vi "Write All Elements GUI.vi"(8 "error in (no error)":errorcluster, 10 "Correction params.":T1={"Background correction"=FALSE, "Hot-pixel correction"=FALSE, "Black image cam. 1"=path "C:/CameraVision/Black images/Black-CameraA-Full.bmp", "Black image cam. 2"=path "C:/CameraVision/Black images/Black-CameraB-Full.bmp", "Y-shift"=0, "X-shift"=0, "Correlation algorithm"=enum."Fixed shift", "Noise treshold"=25.0, "Smoothing algorithm"=enum."Noise tresholding", "2nd image correlation"=FALSE, "Image smoothing"=FALSE, "Background correction method"=enum."Hardware"} {"Noise treshold" min=0 max=255 step=1}, 11 "Correct params in":refnum<class "CV-Correction.lvclass">) -> (0 "error out":errorcluster, 3 "Correct params out":refnum<class "CV-Correction.lvclass">)   [LabVIEW 2013, in "CameraVision.lvlib" / "CV-Correction.lvclass"]
uses:
  CV-Correction.lvclass
  Correction-parameters-gui.ctl
  Smoothing.ctl
  Background-correction.ctl
  CV-Correction.lvclass/CV-Correction.ctl
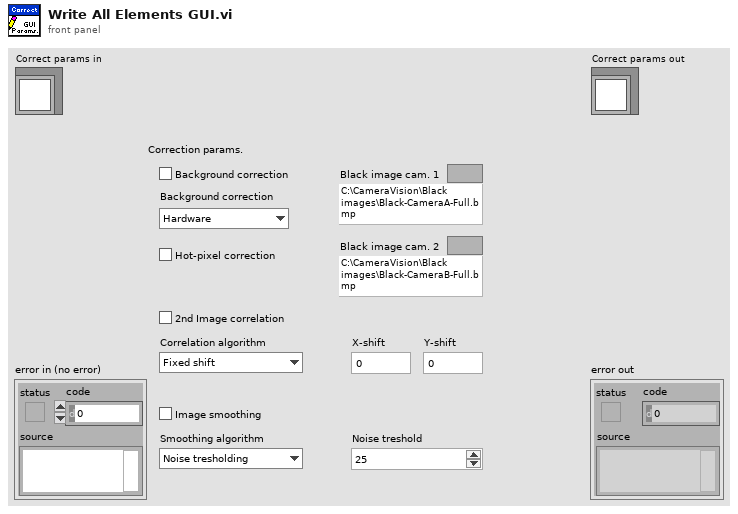
[diagram p1: front panel]
types:
  T1 = typedef "CameraVision.lvlib/CV-Correction.lvclass/Correction-parameters-gui.ctl" = cluster{"Background correction":bool, "Hot-pixel correction":bool, "Black image cam. 1":path, "Black image cam. 2":path, "Y-shift":i32, "X-shift":i32, "Correlation algorithm":enum16{"Fixed shift", "Cross-correlation", "Cross-correlation (5steps)", "Melt-pool center"}, "Noise treshold":sgl, "Smoothing algorithm":T2, "2nd image correlation":bool, "Image smoothing":bool, "Background correction method":T3}
  T2 = typedef "CameraVision.lvlib/CV-Correction.lvclass/Smoothing.ctl" = enum16{"Noise tresholding", "NT+Median filter", "NT+Gaussian filter"}
  T3 = typedef "CameraVision.lvlib/CV-Correction.lvclass/Background-correction.ctl" = enum16{"Hardware", "Software"}
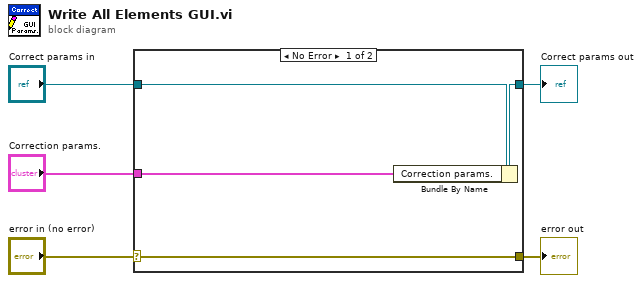
[diagram p0: block diagram]
diagram:
  n1 = case shown="No Error" "error in (no error)" {
    selector: "error in (no error)" -> [w9 w10]
    tunnel: [w9 w10] -> w4
    tunnel: [w7 w11] -> w2
    tunnel: "Correct params in" -> [w8 w11]
    tunnel: "Correction params." -> [w6 _]
    frame No Error {
      n2 = Bundle By Name(cluster=w8, "Correction params."=w6) -> (w7:refnum<class "CV-Correction.lvclass">)
    }
    frame Error {
    }
  }
  "error out" <- w4
  "Correct params out" <- w2
